vi "host test.vi"() -> ()   [LabVIEW 2019]
uses:
  <vilib>/FPGAPlugInAG/myRIO-1900/niLvFpga_Open_myRIO-1900.vi
  <vilib>/rvi/interface/common/dynamic/niFpgaDynamicAddResources.vi
  <vilib>/Utility/error.llb/Error Cluster From Error Code.vi
  <vilib>/rvi/errors/niLvFpgaAdjustHostInterfaceError.vi
  <vilib>/FPGAPlugInAG/Dynamic/niLvFpga_Close_Dynamic.vi
  <vilib>/rvi/interface/nirviOpenFPGA/nirviOpenFPGA.xnode
  FPGA Bitfiles/myrioddstest_FPGATarget_ledtest_Nk9Q8yaQ8CA.lvbitx
  led_test.vi
  <vilib>/rvi/interface/nirviMethod/nirviMethod.xnode
  <vilib>/rvi/interface/nirviCloseFPGA/nirviCloseFPGA.xnode
  <vilib>/FPGAPlugInAG/Dynamic/niLvFpga_WriteFifo_Dynamic.vi
  <vilib>/rvi/errors/niLvFpgaMergeErrorWithErrorCode.vi
panel:
  out "Array":u8[](array[numeric])
  in  "N":u8
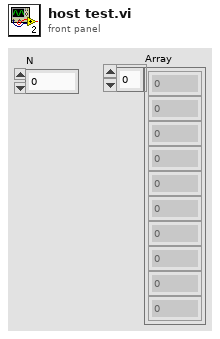
[diagram p1: front panel]
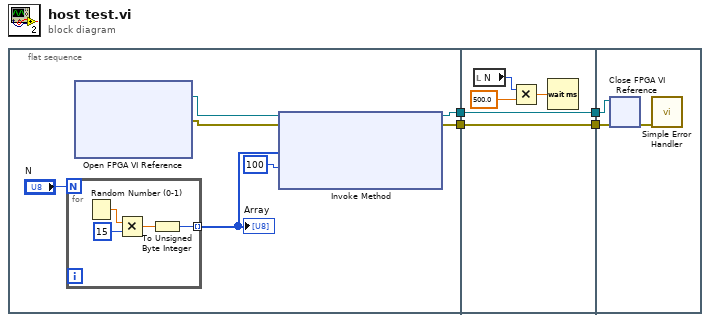
[diagram p0: block diagram]
diagram:
  n1 = flat-sequence {
    tunnel: [w10] -> w3
    tunnel: [w9] -> w1
    tunnel: [w17] -> w4
    tunnel: w3 -> [w17]
    tunnel: [w16] -> w2
    tunnel: w1 -> [w16]
    tunnel: w4 -> [w23]
    tunnel: w2 -> [w22]
    frame #0 {
      n2 = for {
        N: "N" -> [_]
        tunnel: [w12] -> w7 mode=indexing
        n3 = Random Number (0-1)() -> (number: 0 to 1=w15:dbl)
        n4 = Multiply(x=w15, y=u16 15 ("lower bound (0)")) -> (x*y=w13:dbl)
        n5 = To Unsigned Byte Integer(number=w13) -> (unsigned 8bit integer=w12:u8)
      }
      "Array" <- w7
      n6 = xnode "Open FPGA VI Reference"() -> ("FPGA VI Reference Out"=w6:refnum<k20>, "error out"=w5:errorcluster)  [unwired: 2 in]
      n7 = xnode "Invoke Method"("FPGA VI Reference In"=w6, "error in"=w5, "Data"=w7, "Timeout (ms)"=100) -> ("FPGA VI Reference Out"=w10:refnum<k20>, "error out"=w9:errorcluster)  [unwired: 1 out]
    }
    frame #1 {
      n8 = local read "N"() -> (w19:u8)
      n9 = Multiply(x=w19, y=500.0) -> (x*y=w18:dbl)
      n10 = Wait (ms)(milliseconds to wait=w18) -> ()  [unwired: 1 out]
    }
    frame #2 {
      n11 = xnode "Close FPGA VI Reference"("FPGA VI Reference In"=w23, "error in"=w22) -> ("error out"=w21:errorcluster)
      n12 = call <vilib>:"Simple Error Handler.vi"("error in (no error)"=w21) -> ()  [unwired: 4 in, 5 out]
    }
  }
